vi "Get Server State.vi"(8 "error in (no error)":errorcluster, 11 "Template Server in":refnum<class "HVC9.lvclass">) -> (0 "error out":errorcluster, 2 "Server Internal State":T1, 3 "Template Server out":refnum<class "HVC9.lvclass">)   [LabVIEW 2019, in "HVC9.lvlib" / "HVC9.lvclass"]
uses:
  HVC9.lvclass
  typeDefs/Server State Data.ctl
  HVC9.lvclass/HVC9.ctl
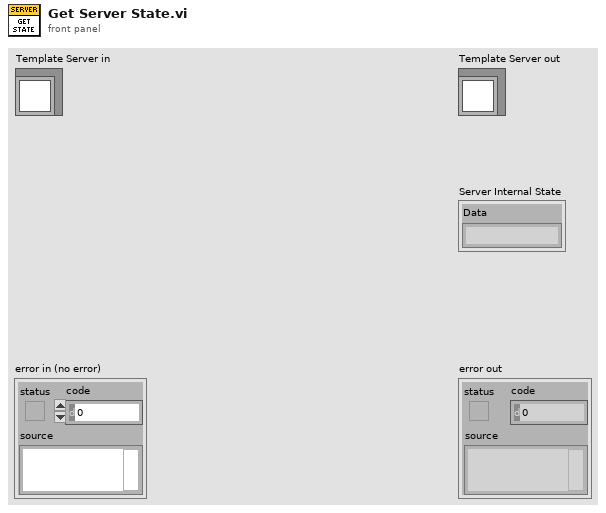
[diagram p1: front panel]
types:
  T1 = typedef "HVC9.lvlib/HVC9.lvclass/Server State Data.ctl" = cluster{"Data":string}
  T2 = typedef "Template Server.lvlib/Template Server.lvclass/Server State Data.ctl" = cluster{"Data":string}
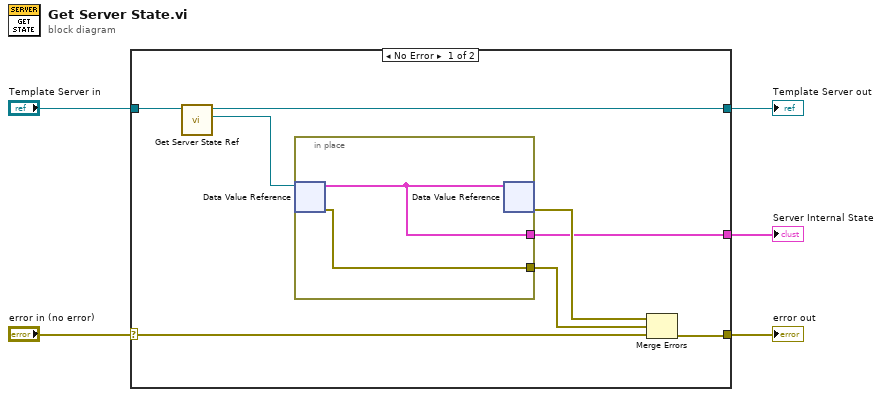
[diagram p0: block diagram]
diagram:
  n1 = case shown="No Error" "error in (no error)" {
    selector: "error in (no error)" -> [w10 w17]
    tunnel: [w7 w17] -> w4
    tunnel: [w12 w16] -> w2
    tunnel: "Template Server in" -> [w13 w16]
    tunnel: [w6 _] -> w1
    frame No Error {
      n2 = call "Get Server State Ref.vi"("Template Server in"=w13) -> ("Server State Ref"=w11:refnum<data-value>, "Template Server out"=w12:refnum<class "HVC9.lvclass">)  [unwired: 9 in]
      n3 = in-place {
        in-place-border: [w15] -> w6
        in-place-border: [w14] -> w8
        n4 = in-place-dvr #1(w11) -> (w15:T2, w14:errorcluster)
        n5 = in-place-dvr #1(w15) -> (w9:errorcluster)  [unwired: 1 out]
      }
      n6 = Merge Errors(w9, w8, w10) -> (w7:errorcluster)
    }
    frame Error {
    }
  }
  "error out" <- w4
  "Template Server out" <- w2
  "Server Internal State" <- w1
